vi "UART Write.vi"(8 "Error In":errorcluster, 9 "Data":u8[](array[numeric]), 10 "UART Channel (0)":u8, 11 "LINX Resource":T1) -> (0 "Error Out":errorcluster, 3 "LINX Resource":T1)   [LabVIEW 2013, in "LVH-LINX.lvlib"]
doc: "Transmit data using the specified UART channel."
uses:
  <vilib>/LabVIEW Hacker/LINX/LVH-LINX.lvlib
  <vilib>/LabVIEW Hacker/LINX/Private/Type Defs/LINX Ref.ctl
  <vilib>/LabVIEW Hacker/LINX/Private/Type Defs/Platform.ctl
  <vilib>/LabVIEW Hacker/LINX/Private/Type Defs/Interface.ctl
  <vilib>/LabVIEW Hacker/LINX/Private/Device/Type Defs/LINX Device Config.ctl
  <vilib>/LabVIEW Hacker/LINX/Private/Device/Type Defs/TCP Config.ctl
  <vilib>/LabVIEW Hacker/LINX/Private/Type Defs/Device Family.ctl
  <vilib>/LabVIEW Hacker/LINX/Private/Type Defs/Peripheral.ctl
  <vilib>/LabVIEW Hacker/LINX/Private/Type Defs/Channel FGV States.ctl
  <vilib>/LabVIEW Hacker/LINX/Private/Device/Device.lvlib
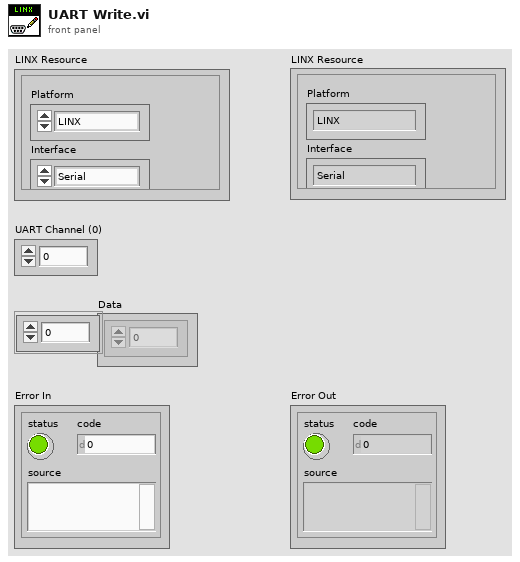
[diagram p1: front panel]
types:
  T1 = typedef "LVH-LINX.lvlib/LINX Ref.ctl" = cluster{"Platform":T2, "Interface":T3, "LINX Device Config":T4}
  T2 = typedef "LVH-LINX.lvlib/Platform.ctl" = enum16{"LINX", "myRIO"}
  T3 = typedef "LVH-LINX.lvlib/Interface.ctl" = enum16{"Serial", "TCP"}
  T4 = typedef "LVH-LINX.lvlib/Device.lvlib/LINX Device Config.ctl" = cluster{"Interface":T3, "COM Port":refnum<visa-resource-name>, "TCP Configuration":T5, "Device Family":T6, "Device ID":u8, "Device Name":string, "TCP Ref":refnum<k5>}
  T5 = typedef "LVH-LINX.lvlib/Device.lvlib/TCP Config.ctl" = cluster{"IP Address":string, "Port":u16}
  T6 = typedef "LVH-LINX.lvlib/Device Family.ctl" = enum8{"National Instruments", "Digilent", "Arduino"}
  T7 = typedef "LVH-LINX.lvlib/Peripheral.ctl" = enum8{"DI", "DO", "AI", "AO", "PWM", "QE", "UART", "I2C", "SPI", "CAN"}
  T8 = typedef "LVH-LINX.lvlib/Channel FGV States.ctl" = enum16{"Initialize", "Get", "Set"}
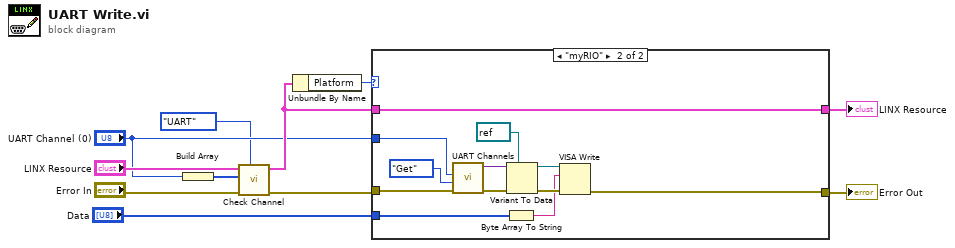
[diagram p0: block diagram]
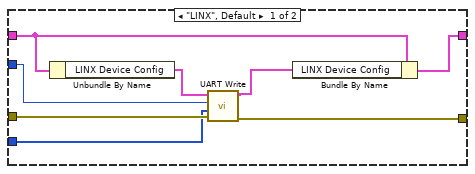
[diagram p2: hidden frame]
diagram:
  n1 = Build Array("UART Channel (0)") -> (w4:u8[])
  n2 = call <vilib>:"Check Channel.vi"("Peripheral"=Peripheral."UART", "Error In"="Error In", "Channels"=w4, "LINX Resource"="LINX Resource") -> ("Error Out"=w5:errorcluster, "LINX Resource"=w6:T1)  [unwired: 5 in, 1 out]
  n3 = Unbundle By Name(w6) -> ("Platform"=w11:T2)
  n4 = case shown="\"myRIO\"" w11 {
    tunnel: w5 -> [w16 w30]
    tunnel: w6 -> [w19 w31]
    tunnel: [w17 w22] -> w10
    tunnel: [w18 w31] -> w9
    tunnel: "UART Channel (0)" -> [w13 w26]
    tunnel: "Data" -> [w12 w20]
    frame "LINX", Default {
      n5 = Unbundle By Name(w19) -> ("LINX Device Config"=w15:T4)
      n6 = call <vilib>:"UART Write.vi"("Error In"=w16, "Data"=w12, "UART Channel"=w13, "LINX Device Config"=w15) -> ("Error Out"=w17:errorcluster, "LINX Device Config"=w14:T4)  [unwired: 6 in]
      n7 = Bundle By Name(cluster=w19, "LINX Device Config"=w14) -> (w18:T1)
    }
    frame "myRIO" {
      n8 = call <vilib>:"UART Channels.vi"("Error In"=w30, "Channel State"=Channel_FGV_States."Get", "Channel Number"=w26) -> ("Error Out"=w29:errorcluster, "UART Channel"=w28:variant)  [unwired: 7 in]
      n9 = Byte Array To String(unsigned byte array=w20) -> (string=w21:string)
      n10 = Variant To Data(error in=w29, type=refnum<visa-resource-name> refnum ("reference"), Variant=w28) -> (data=w23:refnum<visa-resource-name>, error out=w24:errorcluster)
      n11 = VISA Write(VISA resource name=w23, write buffer=w21, error in (no error)=w24) -> (error out=w22:errorcluster)  [unwired: 2 out]
    }
  }
  "Error Out" <- w10
  "LINX Resource" <- w9
